vi "Remove IP Address from CD Path.vi"(11 "CD Path":string) -> (3 "Path":string)   [LabVIEW 2015, in "Diagnostics Addon Shared.lvlib"]
uses:
  Diagnostics Addon Shared.lvlib
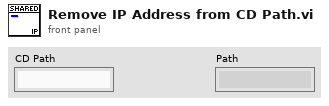
[diagram p1: front panel]
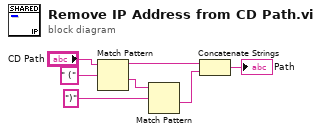
[diagram p0: block diagram]
diagram:
  n1 = Match Pattern(string="CD Path", regular expression=" (") -> (before substring=w5:string, after substring=w3:string)  [unwired: 1 in, 2 out]
  n2 = Match Pattern(string=w3, regular expression=")") -> (after substring=w4:string)  [unwired: 1 in, 3 out]
  n3 = Concatenate Strings(w5, w4) -> (→"Path":string)
